vi "AB_Engine_FindVisitedVI.vi"(10 "path":path, 11 "hash table":variant) -> (0 "index of element":i32, 2 "path out":path, 3 "hash table out":variant)   [LabVIEW 2020]
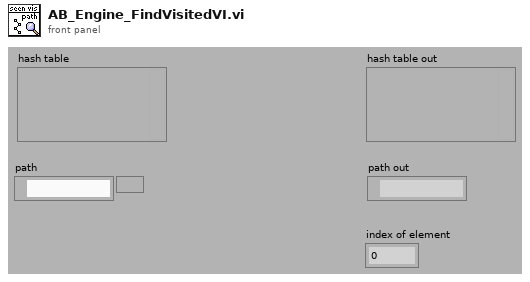
[diagram p1: front panel]
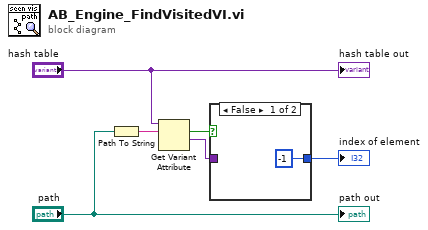
[diagram p0: block diagram]
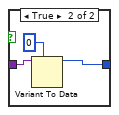
[diagram p2: hidden frame]
diagram:
  n1 = Path To String(path="path") -> (string=w5:string)
  n2 = Get Variant Attribute(Variant="hash table", name=w5) -> (found=w4:bool, value=w3:variant)  [unwired: 2 in, 2 out]
  n3 = case shown="False" w4 {
    tunnel: w3 -> [_ w10]
    tunnel: [-1 ("index of element") w9] -> w2
    frame False {
    }
    frame True {
      n4 = Variant To Data(type=0 ("index of element"), Variant=w10) -> (data=w9:i32)  [unwired: 1 in, 1 out]
    }
  }
  "index of element" <- w2
  "path out" <- "path"
  "hash table out" <- "hash table"
